vi "createViewer.vi"(7 "CommandEvents.lvclass":refnum<class "CommandEvents.lvclass">, 8 "error in (no error)":errorcluster, 9 "SettingsEventsManager.lvclass":refnum<class "SettingsEventsManager.lvclass">, 10 "Path":path, 11 "Tools.lvlib:Settings.lvlib:ConsoleViewer.lvclass":refnum<class "ConsoleViewer.lvclass">) -> (0 "error out":errorcluster, 3 "ConsoleViewer out":refnum<class "ConsoleViewer.lvclass">)   [LabVIEW 2009, in "Views.lvlib" / "ConsoleViewer.lvclass"]
uses:
  ConsoleViewer.lvclass
  Tools/SettingsEventManager/SettingsEventsManager.lvclass
  Tools/CommandProcessor/CommandEvents/CommandEvents.lvclass
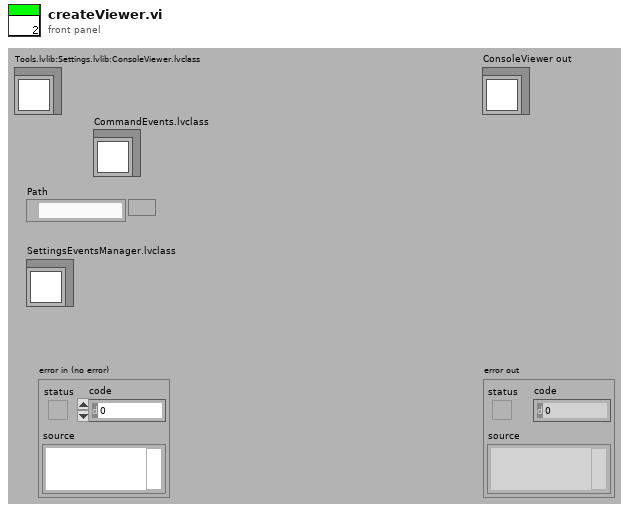
[diagram p1: front panel]
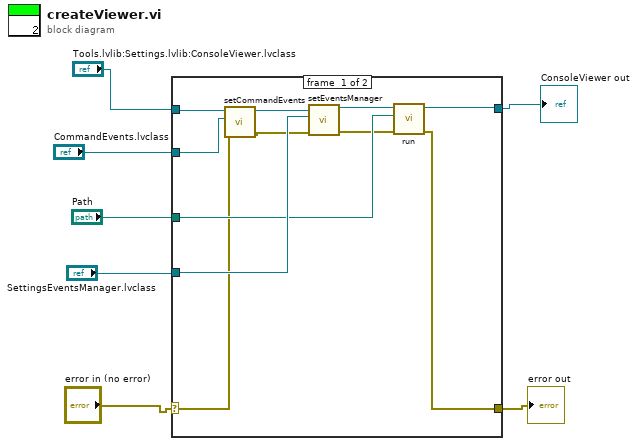
[diagram p0: block diagram]
diagram:
  n1 = case shown="No Error" "error in (no error)" {
    selector: "error in (no error)" -> [w10 w19]
    tunnel: [w14 w19] -> w6
    tunnel: "Tools.lvlib:Settings.lvlib:ConsoleViewer.lvclass" -> [w12 w20]
    tunnel: [w13 w20] -> w4
    tunnel: "SettingsEventsManager.lvclass" -> [w18 _]
    tunnel: "Path" -> [w16 _]
    tunnel: "CommandEvents.lvclass" -> [w11 _]
    frame #0 {
      n2 = call-dynamic "setCommandEvents.vi"("error in (no error)"=w10, "Tools.lvlib:Interpreters.lvlib:CommandEvents.lvclass"=w11, "ConsoleViewer.lvclass in"=w12) -> ("error out"=w9:errorcluster, "ConsoleViewer.lvclass out"=w8:refnum<class "ConsoleViewer.lvclass">)  [unwired: 7 in]
      n3 = call-dynamic "setEventsManager.vi"("error in (no error)"=w9, "Tools.lvlib:Settings.lvlib:SettingsEventsManager.lvclass"=w18, "settingsViewer.lvclass in"=w8) -> ("error out"=w15:errorcluster, "settingsViewer.lvclass out"=w17:refnum<class "ConsoleViewer.lvclass">)  [unwired: 7 in]
      n4 = call-dynamic "run.vi"("error in (no error)"=w15, "Path"=w16, "ConsoleViewer in"=w17) -> ("error out"=w14:errorcluster, "ConsoleViewer out"=w13:refnum<class "ConsoleViewer.lvclass">)  [unwired: 7 in]
    }
    frame #1 {
    }
  }
  "error out" <- w6
  "ConsoleViewer out" <- w4
